vi "Goniometer_Conversion.vi"(1 "Goniometer Output (V)":dbl) -> (0 "Elbow Angle":dbl)   [LabVIEW 2020]
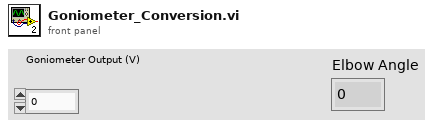
[diagram p1: front panel]
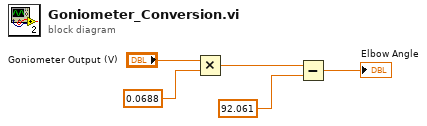
[diagram p0: block diagram]
diagram:
  n1 = Multiply(x="Goniometer Output (V)", y=0.0688 ("x")) -> (x*y=w2:dbl)
  n2 = Subtract(x=w2, y=92.061 ("x")) -> (x-y=→"Elbow Angle":dbl)
